vi "Set Buffer Offsets.vi"(8 "error in (no error)":errorcluster, 9 "inline buffer offset":u64, 10 "string buffer offset":u64, 11 "Buffers in":refnum<class "Buffers.lvclass">) -> (0 "error out":errorcluster, 3 "Buffers out":refnum<class "Buffers.lvclass">)   [LabVIEW 2017, in "DSF Core.lvlib" / "Buffers.lvclass"]
uses:
  Buffers.lvclass
  Buffers.lvclass/Buffers.ctl
  Buffer.lvclass/Buffer.ctl
  Buffer.lvclass
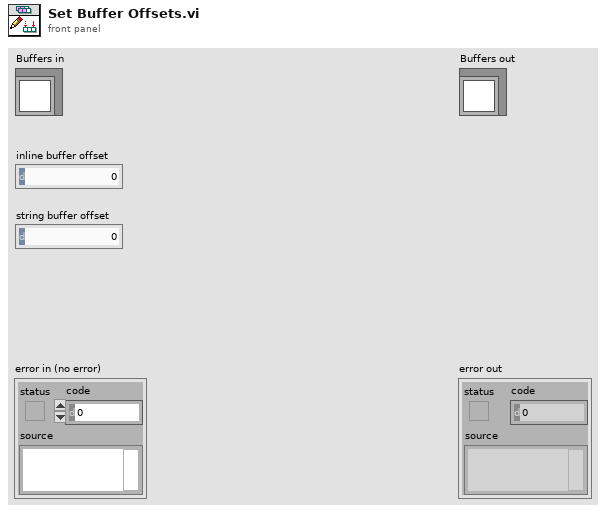
[diagram p1: front panel]
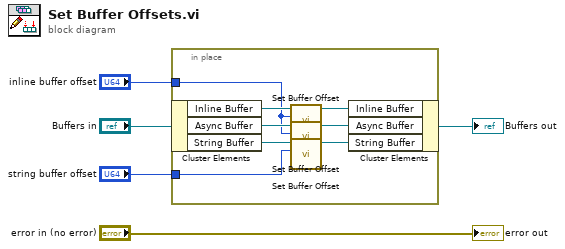
[diagram p0: block diagram]
diagram:
  n1 = in-place {
    in-place-border: "inline buffer offset" -> [w7]
    in-place-border: "string buffer offset" -> [w6]
    n2 = in-place-cluster #1("Buffers in") -> ("Inline Buffer"=w13:refnum<class "Buffer.lvclass">, "Async Buffer"=w12:refnum<class "Buffer.lvclass">, "String Buffer"=w11:refnum<class "Buffer.lvclass">)
    n3 = call "Set Buffer Offset.vi"("buffer offset"=w7, "Buffer in"=w13) -> ("Buffer out"=w10:refnum<class "Buffer.lvclass">)  [unwired: 9 in]
    n4 = call "Set Buffer Offset.vi"("buffer offset"=w7, "Buffer in"=w12) -> ("Buffer out"=w9:refnum<class "Buffer.lvclass">)  [unwired: 9 in]
    n5 = call "Set Buffer Offset.vi"("buffer offset"=w6, "Buffer in"=w11) -> ("Buffer out"=w8:refnum<class "Buffer.lvclass">)  [unwired: 9 in]
    n6 = in-place-cluster #1("Inline Buffer"=w10, "Async Buffer"=w9, "String Buffer"=w8) -> (→"Buffers out":refnum<class "Buffers.lvclass">)
  }
  "error out" <- "error in (no error)"
